vi "Set Header Object Positions.vi"(4 "FP.width":i16, 8 "error in":errorcluster, 10 "label array in":string[](array[string]), 11 "controls[] in":refnum<vi>[](array[refnum])) -> (0 "error out":errorcluster, 2 "label array out":string[](array[string]), 3 "controls[] out":refnum<vi>[](array[refnum]))   [LabVIEW 2018]
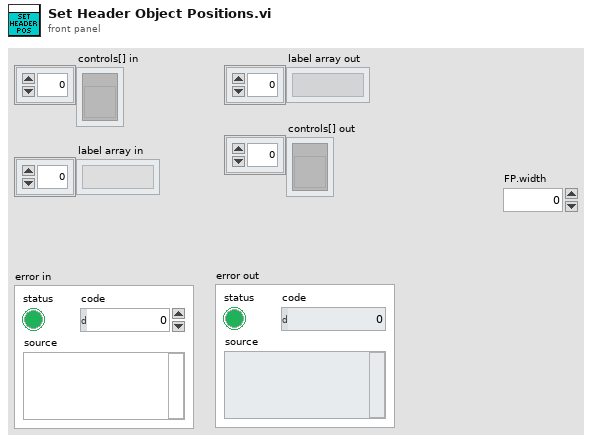
[diagram p1: front panel]
types:
  T1 = typedef "LVRectTypeDef.ctl" = cluster{"Left":i16, "Top":i16, "Right":i16, "Bottom":i16}
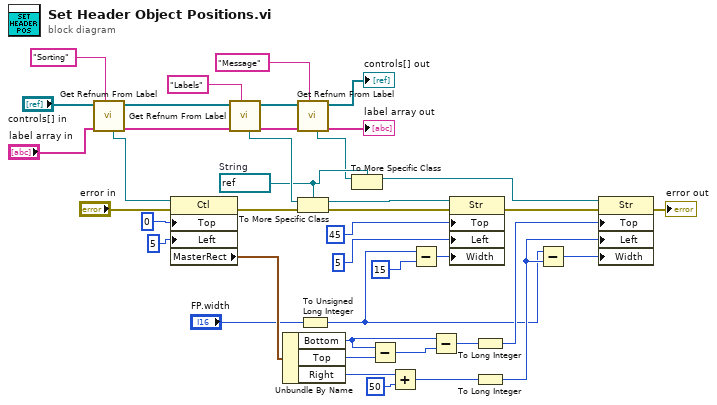
[diagram p0: block diagram]
diagram:
  w9 = refnum<vi> refnum  # String
  n1 = call "Get Refnum From Label.vi"("label"="Sorting" ("element"), "label array in"="label array in", "controls[] in"="controls[] in") -> ("label array out"=w17:string[], "controls[] out"=w16:refnum<vi>[], "refnum out"=w18:refnum<vi>)  [unwired: 6 in]
  n2 = property class="Ctl"(reference=w18, error in="error in", "Top"=0 ("Position:Left"), "Left"=5 ("Position:Top")) -> (error out=w36:errorcluster, "MasterRect"=w29:T1)  [unwired: 1 out]
  n3 = call "Get Refnum From Label.vi"("label"="Labels" ("element"), "label array in"=w17, "controls[] in"=w16) -> ("label array out"=w38:string[], "controls[] out"=w39:refnum<vi>[], "refnum out"=w33:refnum<vi>)  [unwired: 6 in]
  n4 = Unbundle By Name(w29) -> ("Bottom"=w30:i16, "Top"=w24:i16, "Right"=w25:i16)
  n5 = call "Get Refnum From Label.vi"("label"="Message", "label array in"=w38, "controls[] in"=w39) -> ("label array out"=→"label array out":string[], "controls[] out"=→"controls[] out":refnum<vi>[], "refnum out"=w8:refnum<vi>)  [unwired: 6 in]
  n6 = To More Specific Class(target class=w9, reference=w33, error in=w36) -> (specific class reference=w34:refnum<vi>, error out=w37:errorcluster)
  n7 = To Unsigned Long Integer(number="FP.width") -> (unsigned 32bit integer=w3:u32)
  n8 = To More Specific Class(target class=w9, reference=w8) -> (specific class reference=w7:refnum<vi>)  [unwired: 1 in, 1 out]
  n9 = Subtract(x=w30, y=w24) -> (x-y=w31:i16)
  n10 = Add(x=w25, y=i16 50) -> (x+y=w27:i16)
  n11 = Subtract(x=w3, y=u32 15 ("Position:Left")) -> (x-y=w1:u32)
  n12 = Subtract(x=w30, y=w31) -> (x-y=w32:i16)
  n13 = property class="Str"(reference=w34, error in=w37, "Top"=45 ("Position:Top"), "Left"=5 ("Position:Left"), "Width"=w1) -> (error out=w11:errorcluster)  [unwired: 1 out]
  n14 = To Long Integer(number=w32) -> (32bit integer=w26:i32)
  n15 = To Long Integer(number=w27) -> (32bit integer=w6:i32)
  n16 = Subtract(x=w3, y=w6) -> (x-y=w5:u32)
  n17 = property class="Str"(reference=w7, error in=w11, "Top"=w26, "Left"=w6, "Width"=w5) -> (error out=→"error out":errorcluster)  [unwired: 1 out]
